vi "bitarray_to_counts.vi"(1 "16Bit Array":bool[](array[boolean])) -> (0 "Counts":i16)   [LabVIEW 2014]
doc: "Converts 16 bit bit array to counts. The Digitizer stores 12 bits of data in a 16 bits with the 4 least significant bits (LSB) being zero.\nThe conversion conists of converting the 16 bits into an signed 16 bit integer (I16) and dividing by 16 (16=2^4) to account for the 4 zero LSBs."
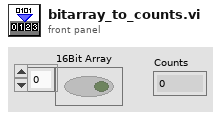
[diagram p1: front panel]
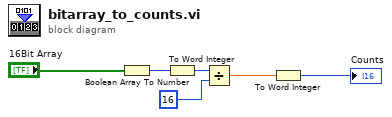
[diagram p0: block diagram]
diagram:
  n1 = Boolean Array To Number(Boolean array="16Bit Array") -> (number=w3:u32)
  n2 = To Word Integer(number=w3) -> (16bit integer=w5:i16)
  n3 = Divide(x=w5, y=16) -> (x/y=w2:dbl)
  n4 = To Word Integer(number=w2) -> (16bit integer=→"Counts":i16)
